vi "Zoom Cache start.vi"(8 "error in (no error)":errorcluster, 10 "Refs":T12, 11 "Loop data in":T1={"TitleCollapse"=refnum, "MouseDownState"=enum."Idle", "RightClickCache"={"Mod"={"Ctrl"=FALSE, "Shift"=FALSE}, "CoordsStart"={"Horizontal"=0, "Vertical"=0}, "CoordsEnd"={"Horizontal"=0, "Vertical"=0}, "PlotAreaBounds"={"Left"=10, "Top"=10, "Right"=0, "Bottom"=0}, "slice"=[]}, "ZoomCache"={"SuppressedPlots"=[], "LeftAxis"={"NeedsRevert?"=FALSE, "Scale Fit"=0, "Range"={"Minimum"=0.0, "Maximum"=0.0, "Increment"=0.0, "Minor Increment"=0.0, "Start"=0.0}}, "RightAxis"={"NeedsRevert?"=FALSE, "Scale Fit"=0, "Range"={"Minimum"=0.0, "Maximum"=0.0, "Increment"=0.0, "Minor Increment"=0.0, "Start"=0.0}}, "Mod"={"Shift"=FALSE}}, "UpdateTime"=0.0, "keyboard"=refnum, "visible?"=FALSE}) -> (0 "error out":errorcluster, 3 "Loop data out":T1={"TitleCollapse"=refnum, "MouseDownState"=enum."Idle", "RightClickCache"={"Mod"={"Ctrl"=FALSE, "Shift"=FALSE}, "CoordsStart"={"Horizontal"=0, "Vertical"=0}, "CoordsEnd"={"Horizontal"=0, "Vertical"=0}, "PlotAreaBounds"={"Left"=10, "Top"=10, "Right"=0, "Bottom"=0}, "slice"=[]}, "ZoomCache"={"SuppressedPlots"=[], "LeftAxis"={"NeedsRevert?"=FALSE, "Scale Fit"=0, "Range"={"Minimum"=0.0, "Maximum"=0.0, "Increment"=0.0, "Minor Increment"=0.0, "Start"=0.0}}, "RightAxis"={"NeedsRevert?"=FALSE, "Scale Fit"=0, "Range"={"Minimum"=0.0, "Maximum"=0.0, "Increment"=0.0, "Minor Increment"=0.0, "Start"=0.0}}, "Mod"={"Shift"=FALSE}}, "UpdateTime"=0.0, "keyboard"=refnum, "visible?"=FALSE})   [LabVIEW 2021, in "RocketPlot.lvlib"]
uses:
  RocketPlot.lvlib
  TypeDefs/Plot UI references.ctl
  Classes/RocketPlotHandle/RocketPlotHandle.lvclass
  <userlib>/bjustice/TipStripOOPanel/Classes/TipPanelHandle/TipPanelHandle.lvclass
  TypeDefs/Plot top row.ctl
  TypeDefs/plot while loop data.ctl
  CollapsePanel/CollapsePanel.lvclass
  TypeDefs/MouseDownState.ctl
  TypeDefs/RightClickCache.ctl
  TypeDefs/RightClickCache PlatMod.ctl
  <vilib>/Utility/miscctls.llb/LVPoint32TypeDef.ctl
  <vilib>/Utility/miscctls.llb/LVRectTypeDef.ctl
  TypeDefs/Slice average.ctl
  TypeDefs/ZoomCache.ctl
  TypeDefs/RangeCache.ctl
  <vilib>/Utility/miscctls.llb/LVRangeTypeDef.ctl
  TypeDefs/ZoomCache PlatMod.ctl
  Plot scale refnum to LUT name.vi
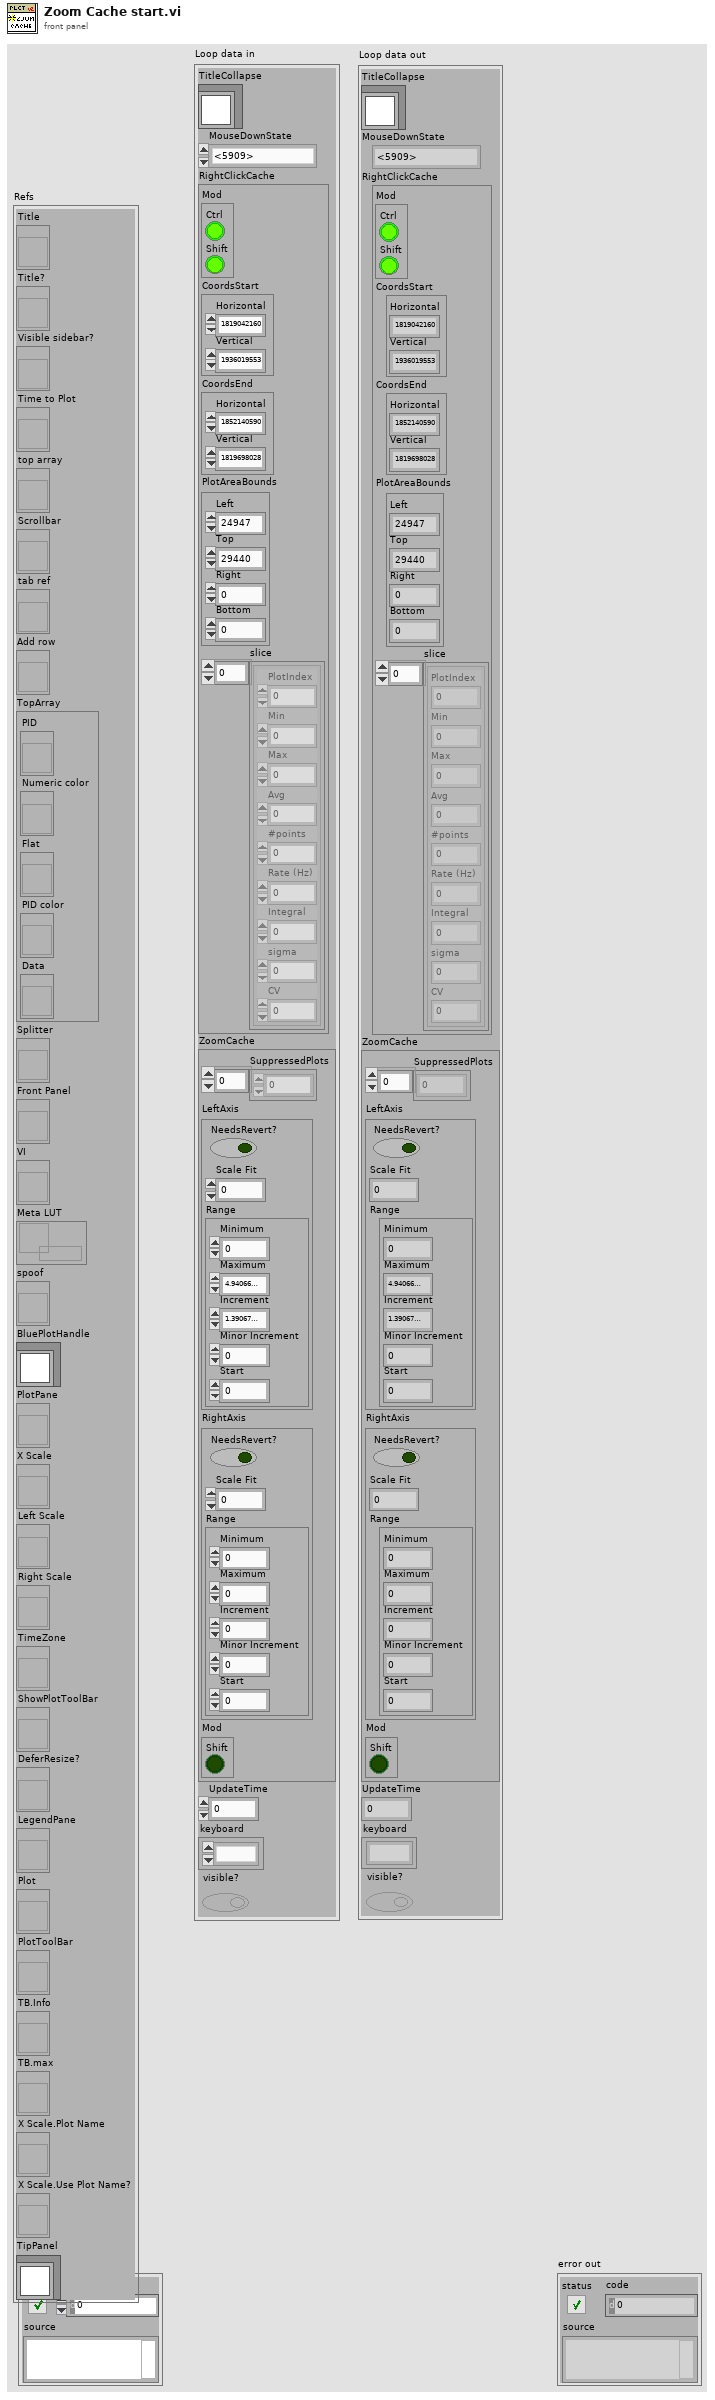
[diagram p1: front panel]
types:
  T1 = typedef "RocketPlot.lvlib/plot while loop data.ctl" = cluster{"TitleCollapse":refnum<class "CollapsePanel.lvclass">, "MouseDownState":T2, "RightClickCache":T3, "ZoomCache":T8, "UpdateTime":dbl, "keyboard":refnum<k1>, "visible?":bool}
  T2 = typedef "RocketPlot.lvlib/MouseDownState.ctl" = enum16{"Idle", "Pan", "Zoom", "Zoom-Post", "RightClick"}
  T3 = typedef "RocketPlot.lvlib/RightClickCache.ctl" = cluster{"Mod":T4, "CoordsStart":T5, "CoordsEnd":T5, "PlotAreaBounds":T6, "slice":T7[]}
  T4 = typedef "RocketPlot.lvlib/RightClickCache PlatMod.ctl" = cluster{"Ctrl":bool, "Shift":bool}
  T5 = typedef "LVPoint32TypeDef.ctl" = cluster{"Horizontal":i32, "Vertical":i32}
  T6 = typedef "LVRectTypeDef.ctl" = cluster{"Left":i16, "Top":i16, "Right":i16, "Bottom":i16}
  T7 = typedef "RocketPlot.lvlib/Slice average.ctl" = cluster{"PlotIndex":i32, "Min":dbl, "Max":dbl, "Avg":dbl, "#points":u32, "Rate (Hz)":dbl, "Integral":dbl, "sigma":dbl, "CV":dbl}
  T8 = typedef "RocketPlot.lvlib/ZoomCache.ctl" = cluster{"SuppressedPlots":i32[], "LeftAxis":T9, "RightAxis":T9, "Mod":T11}
  T9 = typedef "RocketPlot.lvlib/RangeCache.ctl" = cluster{"NeedsRevert?":bool, "Scale Fit":u8, "Range":T10}
  T10 = typedef "LVRangeTypeDef.ctl" = cluster{"Minimum":dbl, "Maximum":dbl, "Increment":dbl, "Minor Increment":dbl, "Start":dbl}
  T11 = typedef "RocketPlot.lvlib/ZoomCache PlatMod.ctl" = cluster{"Shift":bool}
  T12 = typedef "RocketPlot.lvlib/Plot UI references.ctl" = cluster{"Title":refnum<vi>, "Title?":refnum<vi>, "Visible sidebar?":refnum<vi>, "Time to Plot":refnum<vi>, "top array":refnum<vi>, "Scrollbar":refnum<vi>, "tab ref":refnum<vi>, "Add row":refnum<vi>, "TopArray":cluster{"PID":refnum<vi>, "Numeric color":refnum<vi>, "Flat":refnum<vi>, "PID color":refnum<vi>, "Data":refnum<vi>}, "Splitter":refnum<vi>, "Front Panel":refnum<vi>, "VI":refnum<vi>, "Meta LUT":refnum<data-value>, "spoof":refnum<vi>, "BluePlotHandle":refnum<class "RocketPlotHandle.lvclass">, "PlotPane":refnum<vi>, "X Scale":refnum<vi>, "Left Scale":refnum<vi>, "Right Scale":refnum<vi>, "TimeZone":refnum<vi>, "ShowPlotToolBar":refnum<vi>, "DeferResize?":refnum<vi>, "LegendPane":refnum<vi>, "Plot":refnum<vi>, "PlotToolBar":refnum<vi>, "TB.Info":refnum<vi>, "TB.max":refnum<vi>, "X Scale.Plot Name":refnum<vi>, "X Scale.Use Plot Name?":refnum<vi>, "TipPanel":refnum<class "TipPanelHandle.lvclass">}
  T13 = typedef "RocketPlot.lvlib/Plot scale meta JSON.ctl" = cluster{"Type":T14, "Grid Colors:Major Color":u32, "Grid Colors:Minor Color":u32, "Style":u8, "Tick Colors:Tick Color":u32, "Tick Colors:Minor Tick Color":u32, "Format String":string, "State":T15, "AxisFocus":refnum<vi>}
  T14 = typedef "RocketPlot.lvlib/Plot axis.ctl" = enum16{"x axis", "left axis", "right axis"}
  T15 = typedef "RocketPlot.lvlib/Plot scale meta state.ctl" = cluster{"Visible":bool, "Focus":bool, "Multi-Y":bool}
  T16 = typedef "StokePlot.lvlib/Plot top row.ctl" = cluster{"PID":string, "index":i32, "PID color":u32, "right axis?":bool, "Flatline?":bool, "Numeric color":u32, "Data":string, "Flat":string}
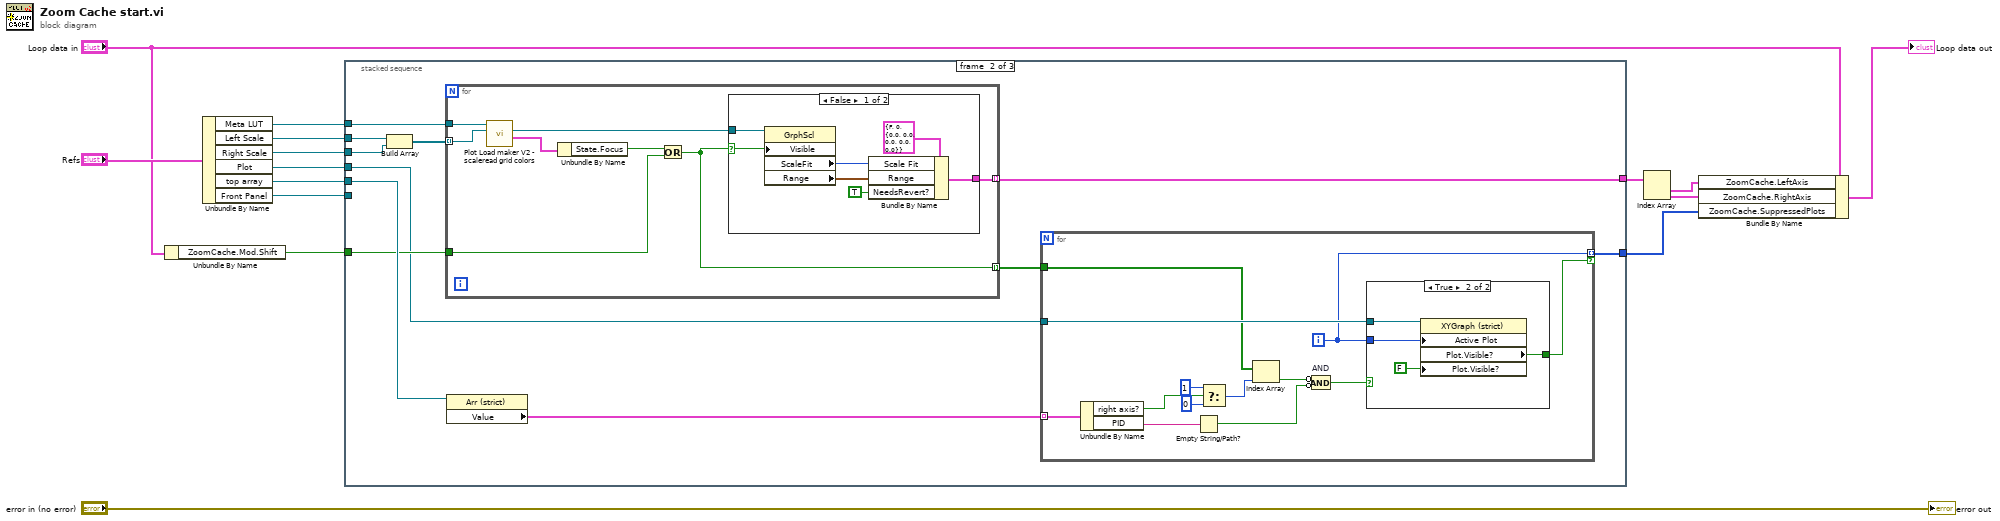
[diagram p0: block diagram]
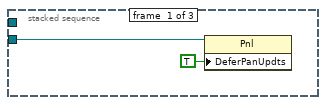
[diagram p2: hidden frame]
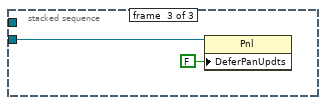
[diagram p5: hidden frame]
diagram:
  n1 = Unbundle By Name("Loop data in") -> ("ZoomCache.Mod.Shift"=w5:bool)
  n2 = Unbundle By Name("Refs") -> ("Meta LUT"=w13:refnum<data-value>, "Left Scale"=w12:refnum<vi>, "Right Scale"=w11:refnum<vi>, "Plot"=w4:refnum<vi>, "top array"=w7:refnum<vi>, "Front Panel"=w1:refnum<vi>)
  n3 = stacked-sequence {
    tunnel: w13 -> [_ w28 _]
    tunnel: w12 -> [_ w27 _]
    tunnel: w11 -> [_ w26 _]
    tunnel: [_ w24 _] -> w10
    tunnel: w7 -> [_ w23 _]
    tunnel: [_ w20 _] -> w6
    tunnel: w5 -> [_ w19 _]
    tunnel: w4 -> [_ w18 _]
    tunnel: w1 -> [w16 _ w61]
    frame #0 {
      n4 = property class="Pnl"(reference=w16, "DeferPanUpdts"=TRUE ("Defer Panel Updates")) -> ()  [unwired: 1 in, 2 out]
    }
    frame #1 {
      n5 = Build Array(w27, w26) -> (w25:refnum<vi>[])
      n6 = for {
        tunnel: w28 -> [w36]
        tunnel: w25 -> [w34] mode=indexing
        tunnel: [w33] -> w24 mode=indexing
        tunnel: [w29] -> w21 mode=indexing
        tunnel: w19 -> [w30]
        n7 = call "Plot Load maker V2 - scaleread grid colors.vi"("Scale reference"=w34, "Meta LUT"=w36) -> ("Scale LUT meta"=w35:T13, "Scale reference"=w32:refnum<vi>)  [unwired: 6 in, 2 out]
        n8 = Unbundle By Name(w35) -> ("State.Focus"=w31:bool)
        n9 = Or(x=w31, y=w30) -> (x .or. y?=w29:bool)
        n10 = case shown="False" w29 {
          selector: w29 -> [w37 _]
          tunnel: [w40 _] -> w33
          tunnel: w32 -> [w38 _]
          frame False {
            n11 = property class="GrphScl"(reference=w38, "Visible"=w37) -> ("ScaleFit"=w42:u8, "Range"=w41:T10)  [unwired: 1 in, 2 out]
            n12 = Bundle By Name(cluster=T9 {"NeedsRevert?"=FALSE, "Scale Fit"=0, "Range"={"Minimum"=0.0, "Maximum"=0.0, "Increment"=0.0, "Minor Increment"=0.0, "Start"=0.0}} ("Cluster"), "Scale Fit"=w42, "Range"=w41, "NeedsRevert?"=TRUE) -> (w40:T9)
          }
          frame True {
          }
        }
      }
      n13 = property class="Arr (strict)"(reference=w23) -> ("Value"=w22:T16[])  [unwired: 1 in, 2 out]
      n14 = for {
        tunnel: w22 -> [w56] mode=indexing
        tunnel: w18 -> [w55]
        tunnel: w21 -> [w53]
        tunnel: [w46] -> w20 mode=indexing if=w44
        i -> [w46]
        n15 = Unbundle By Name(w56) -> ("right axis?"=w54:bool, "PID"=w49:string)
        n16 = Empty String/Path?(string/path=w49) -> (empty?=w47:bool)
        n17 = Select(t=1 ("index"), s=w54, f=0 ("index")) -> (s? t:f=w50:i32)
        n18 = Index Array(array=w53, index=w50) -> (element=w48:bool)
        n19 = Compound Arithmetic op=AND "AND"(invert w48, invert w47) -> (w45:bool)
        n20 = case shown="True" w45 {
          tunnel: w55 -> [_ w60]
          tunnel: w46 -> [_ w59]
          tunnel: [_ w57] -> w44
          frame False {
          }
          frame True {
            n21 = property class="XYGraph (strict)"(reference=w60, "Active Plot"=w59, "Plot.Visible?"=FALSE ("Plot.Visible")) -> ("Plot.Visible?"=w57:bool)  [unwired: 1 in, 2 out]
          }
        }
      }
    }
    frame #2 {
      n22 = property class="Pnl"(reference=w61, "DeferPanUpdts"=FALSE ("Defer Panel Updates")) -> ()  [unwired: 1 in, 2 out]
    }
  }
  n23 = Index Array(array=w10) -> (element #1=w9:T9, element #2=w8:T9)  [unwired: 2 in]
  n24 = Bundle By Name(cluster="Loop data in", "ZoomCache.LeftAxis"=w9, "ZoomCache.RightAxis"=w8, "ZoomCache.SuppressedPlots"=w6) -> (→"Loop data out":T1)
  "error out" <- "error in (no error)"
